vi "test_v2.vi"() -> ()   [LabVIEW 2019]
uses:
  class/mqtt/mqttTypedef/mqttBroker.ctl
  class/mqtt/mqttTypedef/mqttConnectionFlags.ctl
  class/mqtt/mqttTypedef/mqttWillInformation.ctl
  class/mqtt/mqttConfigFunction.ctl
  class/mqtt/mqttTXqueue/mqttTXdataQueueFunction.ctl
  class/mqtt/mqttTXqueue/mqttRXsubscriptionEventFunction.ctl
  class/mqtt/mqtt.lvclass
panel:
  in  "connect":bool
  in  "quit":bool
  in  "Start":bool
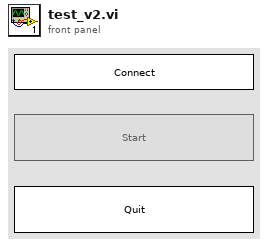
[diagram p1: front panel]
types:
  T1 = typedef "mqtt.lvclass/mqttConfigFunction.ctl" = enum16{"init", "deinit", "set", "get"}
  T2 = typedef "mqttWillInformation.ctl" = cluster{"User Name":string, "Password":string}
  T3 = typedef "mqttConnectionFlags.ctl" = cluster{"reserved":bool, "clean session":bool, "will flag":bool, "willQOS":enum8{"At most once", "At least once", "Exactly once", "Reserved"}, "will retain":bool, "password":bool, "user name":bool}
  T4 = typedef "mqttBroker.ctl" = cluster{"address":string, "port":u16, "connTimeout":i32, "writeTimeout":i32, "readTimeout":i32, "subTimeout":i32}
  T5 = enum8{"Enabled", "Disabled", "Disabled and Grayed Out"}
  T6 = typedef "mqttRXsubscriptionEventFunction.ctl" = enum16{"init", "deinit", "getEventRef", "event"}
  T7 = typedef "mqttTXdataQueueFunction.ctl" = enum16{"init", "deinit", "getQueue", "enqueue"}
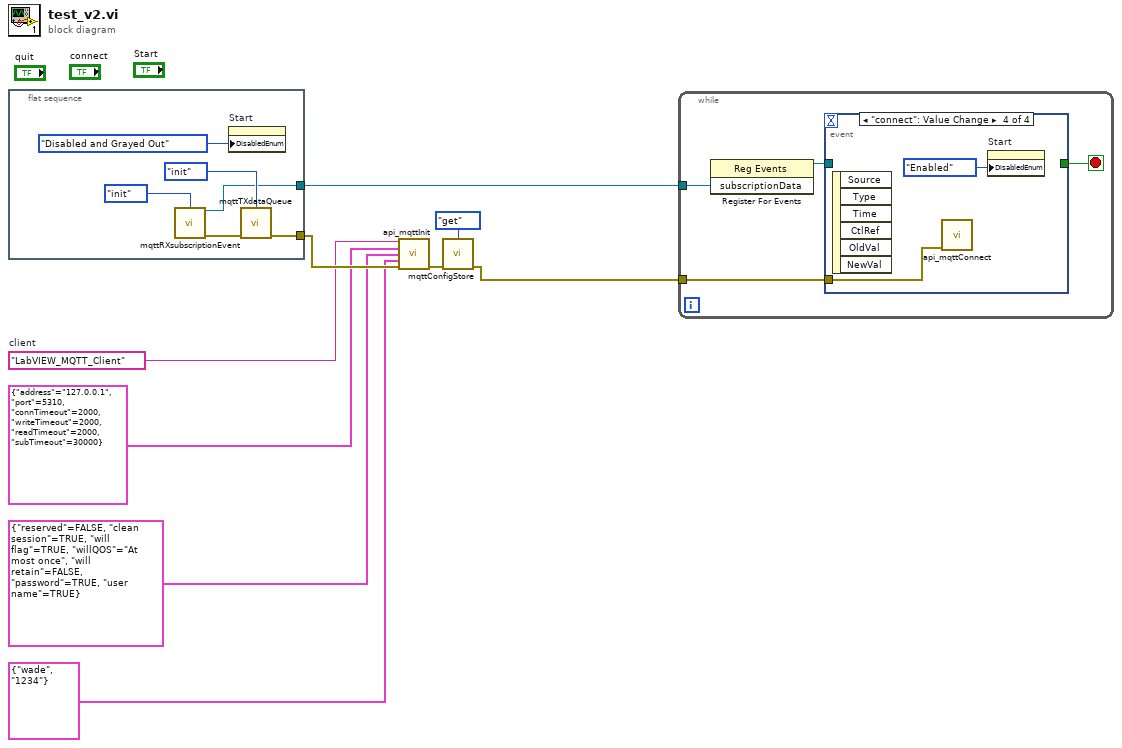
[diagram p0: block diagram]
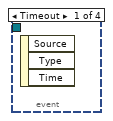
[diagram p2: hidden frame]
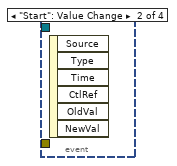
[diagram p3: hidden frame]
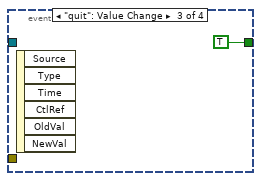
[diagram p4: hidden frame]
diagram:
  w5 = "LabVIEW_MQTT_Client"  # client
  n1 = flat-sequence {
    tunnel: [w14] -> w7
    tunnel: [w11] -> w9
    frame #0 {
      n2 = call "mqttRXsubscriptionEvent.vi"("function"=mqttRXsubscriptionEventFunction."init") -> ("subscriptionData"=w11:refnum<user-event>, "error out"=w13:errorcluster)  [unwired: 13 in]
      n3 = property on="Start" class="Bool"("DisabledEnum"=T5."Disabled and Grayed Out" ("Disabled")) -> ()  [unwired: 2 in, 2 out]
      n4 = call "mqttTXdataQueue.vi"("function"=mqttTXdataQueueFunction."init", "error in (no error)"=w13) -> ("error out"=w14:errorcluster)  [unwired: 12 in, 1 out]
    }
  }
  n5 = call "api_mqttInit.vi"("client"=w5, "broker"=T4 {"address"="127.0.0.1", "port"=5310, "connTimeout"=2000, "writeTimeout"=2000, "readTimeout"=2000, "subTimeout"=30000}, "connFlags"=T3 {"reserved"=FALSE, "clean session"=TRUE, "will flag"=TRUE, "willQOS"=enum."At most once", "will retain"=FALSE, "password"=TRUE, "user name"=TRUE}, "User Info"=T2 {"User Name"="wade", "Password"="1234"}, "error in (no error)"=w7) -> ("error out"=w6:errorcluster)  [unwired: 10 in]
  n6 = call "mqttConfigStore.vi"("function"=mqttConfigFunction."get", "error in (no error)"=w6) -> ("error out"=w1:errorcluster)  [unwired: 12 in, 1 out]
  n7 = while {
    tunnel: w9 -> [w18]
    tunnel: w1 -> [w16]
    stop <- w17 stop-if-true
    n8 = register-events(w18) -> (reference out=w19:refnum<event-registration>)  [unwired: 2 in, 1 out]
    n9 = event shown="[3] \"connect\": Value Change" {
      selector: _ -> [_ _ _ _]
      dyn-events: _ -> [_ _ _ _]
      timeout: _ -> [_ _ _ _]
      tunnel: w19 -> [_ _ _ _]
      tunnel: [_ _ TRUE _] -> w17
      tunnel: w16 -> [_ _ _ w21]
      event Timeout {
        n10 = event-data() -> ()  [unwired: 1 in, 3 out]
      }
      event "Start": Value Change {
        n11 = event-data() -> ()  [unwired: 1 in, 6 out]
      }
      event "quit": Value Change {
        n12 = event-data() -> ()  [unwired: 1 in, 6 out]
      }
      event "connect": Value Change {
        n13 = event-data() -> ()  [unwired: 1 in, 6 out]
        n14 = call "api_mqttConnect.vi"("error in (no error)"=w21) -> ()  [unwired: 11 in, 4 out]
        n15 = property on="Start" class="Bool"("DisabledEnum"=T5."Enabled" ("Disabled")) -> ()  [unwired: 2 in, 2 out]
      }
    }
  }
